vi "List Platform Applications Recursive.vi"(8 "error in (no error)":errorcluster, 9 "NextToken":string, 10 "Region":T1, 11 "AWS Credentials":T2) -> (0 "error out":errorcluster, 3 "Topics out":refnum<class "Platform Application.lvclass">[](array[class]))   [LabVIEW 2015, in "NI_AWS_SNS.lvlib" / "Platform Application.lvclass"]
uses:
  Platform Application.lvclass
  Core/HTTP Request/AWS Credentials.ctl
  Core/HTTP Request/Region.ctl
  Core/HTTP Request/Request Options.ctl
  Core/HTTP Request/Name Value Pair.ctl
  Core/HTTP Request/HTTP Request.lvclass/HTTP Request.ctl
  Core/ARN/ARN.lvclass/ARN.ctl
  Core/ARN/Write ARN.vi
  Core/HTTP Request/Write Credentials.vi
  Core/HTTP Request/Write Region.vi
  Core/HTTP Request/Write Service.vi
  Core/HTTP Request/Write Verify Server.vi
  Core/HTTP Request/HTTP Request.lvclass
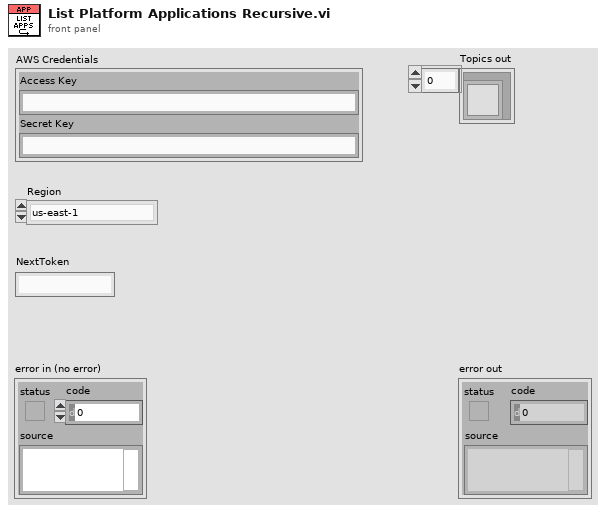
[diagram p1: front panel]
types:
  T1 = typedef "NI_AWS_Core.lvlib/HTTP Request.lvclass/Region.ctl" = enum16{"us-east-1", "us-east-2", "us-west-1", "us-west-2", "ap-northeast-1", "ap-northeast-2", "ap-southeast-1", "ap-southeast-2", "ca-central-1", "eu-central-1", "eu-west-1", "eu-west-2", "sa-east-1"}
  T2 = typedef "NI_AWS_Core.lvlib/HTTP Request.lvclass/AWS Credentials.ctl" = cluster{"Access Key":string, "Secret Key":string}
  T3 = typedef "NI_AWS_Core.lvlib/HTTP Request.lvclass/Name Value Pair.ctl" = cluster{"name":string, "value":string}
  T4 = typedef "NI_AWS_Core.lvlib/HTTP Request.lvclass/Request Options.ctl" = cluster{"request headers":T3[], "request parameters":T3[], "request body":string}
  T5 = typedef "NI_AWS_Core.lvlib/HTTP Request.lvclass/Response.ctl" = cluster{"Headers":string, "Body":string}
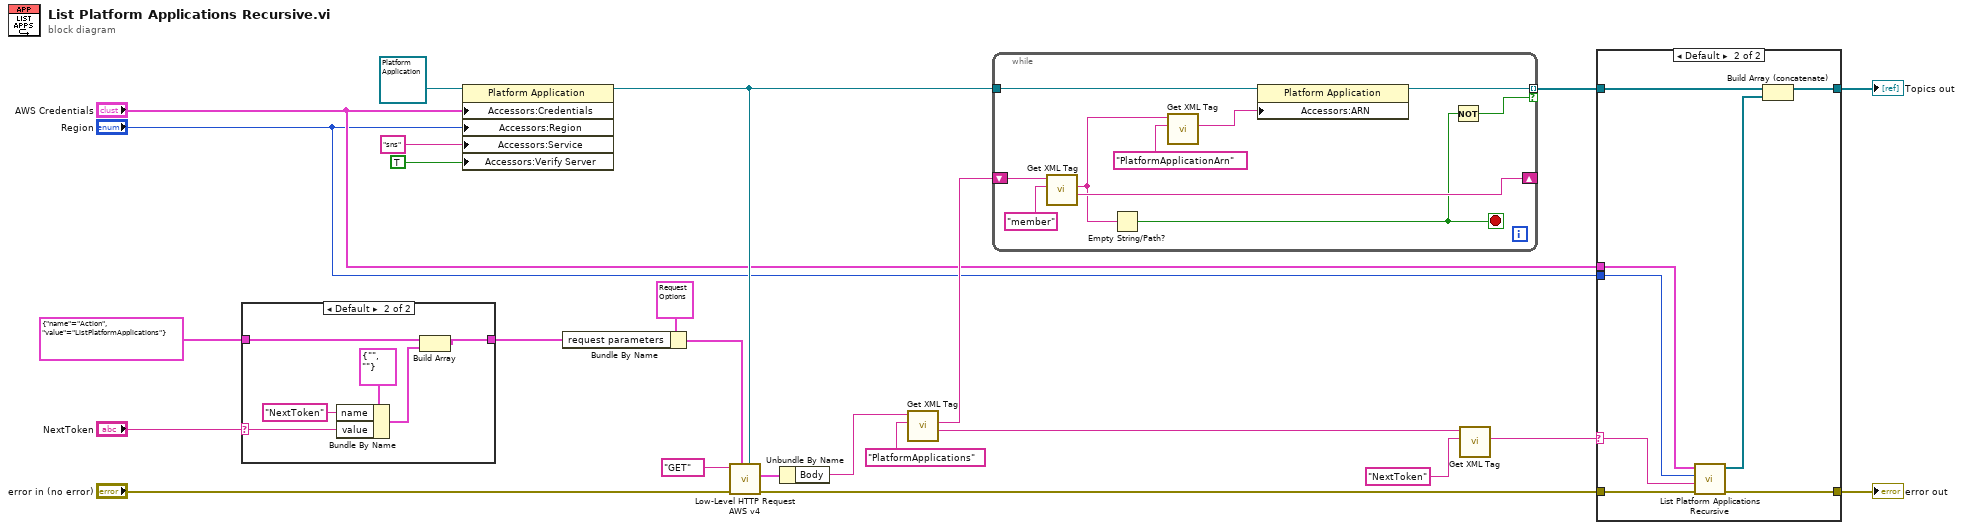
[diagram p0: block diagram]
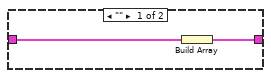
[diagram p2: hidden frame]
diagram:
  n1 = case shown="Default" "NextToken" {
    selector: "NextToken" -> [_ w27]
    tunnel: T3 {"name"="Action", "value"="ListPlatformApplications"} ("Cluster") -> [w26 w32]
    tunnel: [w25 w28] -> w13
    frame "" {
      n2 = Build Array(w26) -> (w25:T3[])
    }
    frame Default {
      n3 = Bundle By Name(cluster=T3 {"name"="", "value"=""} ("element"), "name"="NextToken", "value"=w27) -> (w29:T3)
      n4 = Build Array(w32, w29) -> (w28:T3[])
    }
  }
  n5 = property class="Platform Application"(reference=refnum<class "Platform Application.lvclass"> refnum ("SNS"), "Accessors:Credentials"="AWS Credentials", "Accessors:Region"="Region", "Accessors:Service"="sns" ("Service"), "Accessors:Verify Server"=TRUE ("Verify Server")) -> (reference out=w4:refnum<class "Platform Application.lvclass">)  [unwired: 1 in, 1 out]
  n6 = Bundle By Name(cluster=T4 {"request headers"=[], "request parameters"=[{"name"="Action", "value"="ListQueues"}], "request body"=""} ("Request Options"), "request parameters"=w13) -> (w18:T4)
  n7 = call "Low-Level HTTP Request AWS v4.vi"("AWS Core"=w4, "Request Options"=w18, "error in (no error)"="error in (no error)", "HTTP-Verb"="GET") -> ("error out"=w12:errorcluster, "Response"=w17:T5)  [unwired: 5 in, 1 out]
  n8 = Unbundle By Name(w17) -> ("Body"=w6:string)
  n9 = call "Get XML Tag.vi"("Tag name"="PlatformApplications", "XML String in"=w6) -> ("Remaining string"=w5:string, "Tag value"=w7:string)  [unwired: 5 in, 3 out]
  n10 = while {
    shift-right: [w41] -> _
    shift-left: w7 -> [w42]
    tunnel: w4 -> [w39]
    tunnel: [w34] -> w3 mode=indexing if=w37
    stop <- w38 stop-if-true
    n11 = call "Get XML Tag.vi"("Tag name"="member", "XML String in"=w42) -> ("Remaining string"=w41:string, "Tag value"=w35:string)  [unwired: 5 in, 3 out]
    n12 = Empty String/Path?(string/path=w35) -> (empty?=w38:bool)
    n13 = call "Get XML Tag.vi"("Tag name"="PlatformApplicationArn", "XML String in"=w35) -> ("Tag value"=w33:string)  [unwired: 5 in, 4 out]
    n14 = property class="Platform Application"(reference=w39, "Accessors:ARN"=w33) -> (reference out=w34:refnum<class "Platform Application.lvclass">)  [unwired: 1 in, 1 out]
    n15 = Not(x=w38) -> (.not. x?=w37:bool)
  }
  n16 = call "Get XML Tag.vi"("Tag name"="NextToken", "XML String in"=w5) -> ("Tag value"=w10:string)  [unwired: 5 in, 4 out]
  n17 = case shown="Default" w10 {
    selector: w10 -> [_ w50]
    tunnel: w12 -> [w44 w52]
    tunnel: [w44 w51] -> w11
    tunnel: w3 -> [w43 w47]
    tunnel: [w43 w45] -> w9
    tunnel: "AWS Credentials" -> [_ w49]
    tunnel: "Region" -> [_ w48]
    frame "" {
    }
    frame Default {
      n18 = call "List Platform Applications Recursive.vi"("error in (no error)"=w52, "NextToken"=w50, "Region"=w48, "AWS Credentials"=w49) -> ("error out"=w51:errorcluster, "Topics out"=w46:refnum<class "Platform Application.lvclass">[])  [unwired: 6 in]
      n19 = Build Array (concatenate)(w47, w46) -> (w45:refnum<class "Platform Application.lvclass">[])
    }
  }
  "error out" <- w11
  "Topics out" <- w9
